vi "Create Bus Log File.vi"(11 "Project Folder":path) -> (0 "error out":errorcluster, 1 "Continue":bool, 2 "Status":string, 3 "Byte Stream File out":refnum<file>)   [LabVIEW 2019, in "CAN Stream Support Workspace Shared.lvlib"]
uses:
  CAN Stream Support Workspace Shared.lvlib
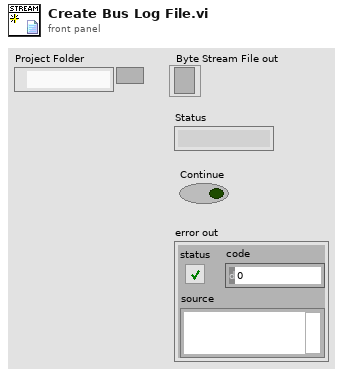
[diagram p1: front panel]
types:
  T1 = enum16{"open", "replace", "create", "open or create", "replace or create", "replace or create with confirmation"}
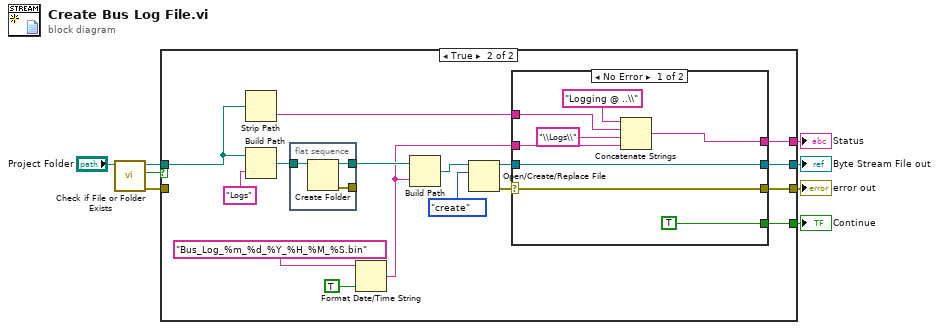
[diagram p0: block diagram]
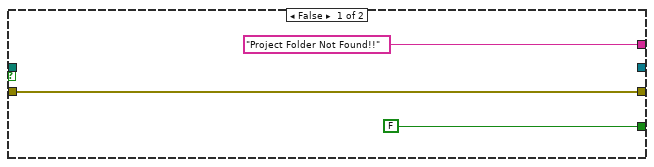
[diagram p2: hidden frame]
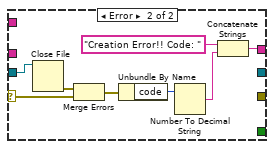
[diagram p3: hidden frame]
diagram:
  n1 = call <vilib>:"Check if File or Folder Exists.vi"("path"="Project Folder") -> ("error out"=w8:errorcluster, "file or folder exists?"=w7:bool, "dup path"=w6:path)  [unwired: 8 in]
  n2 = case shown="True" w7 {
    tunnel: [w10 w26] -> w1
    tunnel: [_ w25] -> w2
    tunnel: [FALSE w23] -> w3
    tunnel: ["Project Folder Not Found!!" w17] -> w4
    tunnel: w6 -> [_ w12]
    tunnel: w8 -> [w10 _]
    frame False {
    }
    frame True {
      n3 = Strip Path(path=w12) -> (name=w13:string)  [unwired: 1 out]
      n4 = Build Path(base path=w12, name or relative path="Logs") -> (appended path=w15:path)
      n5 = flat-sequence {
        tunnel: w15 -> [w30]
        tunnel: [w29] -> _
        tunnel: [w28] -> w19
        frame #0 {
          n6 = Create Folder(path (use dialog)=w30) -> (created path=w28:path, error out=w29:errorcluster)  [unwired: 2 in, 1 out]
        }
      }
      n7 = Format Date/Time String(time format string (%c)="Bus_Log_%m_%d_%Y_%H_%M_%S.bin", UTC format=TRUE) -> (date/time string=w14:string)  [unwired: 1 in]
      n8 = Build Path(base path=w19, name or relative path=w14) -> (appended path=w18:path)
      n9 = Open/Create/Replace File(file path (use dialog)=w18, operation (0:open)=T1."create") -> (refnum out=w27:refnum<file>, error out=w24:errorcluster)  [unwired: 4 in, 1 out]
      n10 = case shown="No Error" w24 {
        selector: w24 -> [w37 w44]
        tunnel: w27 -> [w36 w46]
        tunnel: [w37 _] -> w26
        tunnel: [w36 _] -> w25
        tunnel: [TRUE _] -> w23
        tunnel: [w34 w39] -> w17
        tunnel: w14 -> [w31 _]
        tunnel: w13 -> [w33 _]
        frame No Error {
          n11 = Concatenate Strings("Logging @ ..\\" ("string"), w33, "\\Logs\\" ("string"), w31) -> (w34:string)
        }
        frame Error {
          n12 = Close File(refnum=w46) -> (error out=w45:errorcluster)  [unwired: 1 in, 1 out]
          n13 = Merge Errors(w45, w44) -> (w43:errorcluster)
          n14 = Unbundle By Name(w43) -> ("code"=w42:i32)
          n15 = Number To Decimal String(number=w42) -> (decimal integer string=w41:string)  [unwired: 1 in]
          n16 = Concatenate Strings("Creation Error!! Code: ", w41) -> (w39:string)
        }
      }
    }
  }
  "Status" <- w4
  "Continue" <- w3
  "Byte Stream File out" <- w2
  "error out" <- w1
